vi "Calculate Particle Scores2.vi"(10 "Sorted Data":dbl[][](array[numeric])) -> (3 "Scores":T1[](array[typedef]))   [LabVIEW 2019]
doc: "Calculate scores based on the particle measurements. Calculated scores are for aspect ratio, area to convex hull area, and moment of inertia. These scores range between 0 and 100 and can be used to categorize particles as targets and non-targets."
uses:
  Target Fields.ctl
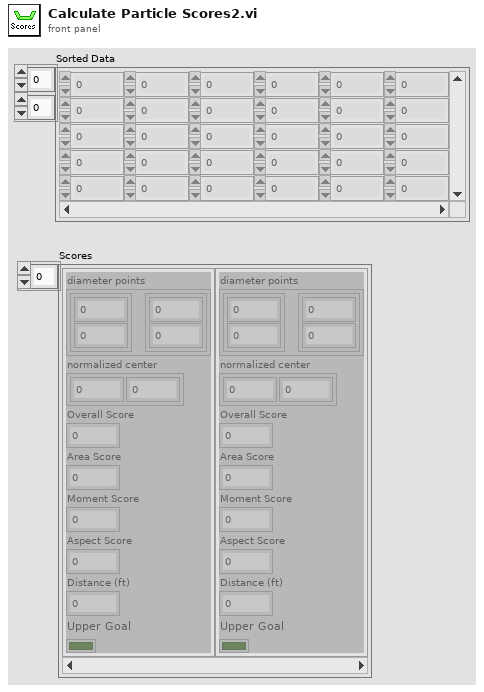
[diagram p1: front panel]
types:
  T1 = typedef "Target Fields.ctl" = cluster{"diameter points":cluster{"first point":cluster{"x":dbl, "y":dbl}, "projected point":cluster{"x":dbl, "y":dbl}}, "normalized center":cluster{"x":dbl, "y":dbl}, "Overall Score":dbl, "Area Score":dbl, "Moment Score":dbl, "Aspect Score":dbl, "Distance (ft)":dbl, "Upper Goal":bool}
  T2 = cluster{cluster{"Numeric":dbl, "Numeric":dbl}, cluster{"Numeric":dbl, "Numeric":dbl}}
  T3 = cluster{"first point":cluster{"x":dbl, "y":dbl}, "projected point":cluster{"x":dbl, "y":dbl}}
  T4 = cluster{cluster{"first point":cluster{"x":dbl, "y":dbl}, "projected point":cluster{"x":dbl, "y":dbl}}, "first point":cluster{"x":dbl, "y":dbl}, dbl, "Score":dbl, "Score":dbl, "Score":dbl, dbl, bool}
  T5 = cluster{cluster{cluster{"Numeric":dbl, "Numeric":dbl}, cluster{"Numeric":dbl, "Numeric":dbl}}, "first point":cluster{"x":dbl, "y":dbl}, dbl, "Score":dbl, "Score":dbl, "Score":dbl, dbl, bool}
  T6 = cluster{cluster{"first point":cluster{"Numeric":dbl, "Numeric":dbl}, "projected point":cluster{"Numeric":dbl, "Numeric":dbl}}, "first point":cluster{"x":dbl, "y":dbl}, dbl, "Score":dbl, "Score":dbl, "Score":dbl, dbl, bool}
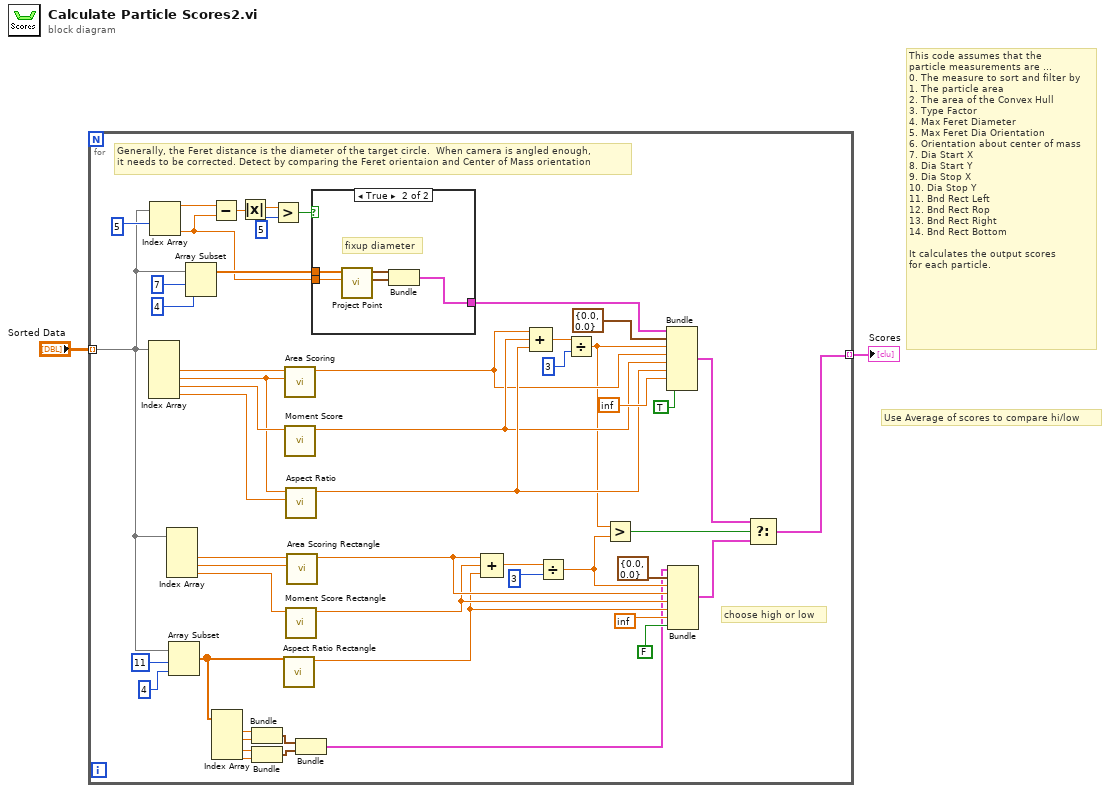
[diagram p0: block diagram]
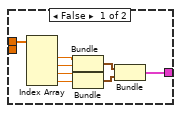
[diagram p2: hidden frame]
diagram:
  # "Use Average of scores to compare hi/low"
  # "This code assumes that the\nparticle measurements are ...\n0. The measure to sort and filter by\n1. The particle area\n2. The area of the Convex Hull\n3. Type Factor\n4. Max Feret Diameter\n5. Max Feret Dia Orientation\n6. Orientation about center of mass\n7. Dia Start X\n8. Dia Start Y\n9. Dia Stop X\n10. Dia Stop Y\n11. Bnd Rect Left\n12. Bnd Rect Rop\n13. Bnd Rect Right\n14. Bnd Rect Bottom\n\nIt calculates the output scores\nfor each particle."
  n1 = for {
    tunnel: "Sorted Data" -> [w27] mode=indexing
    tunnel: [w18] -> w1 mode=indexing
    # "choose high or low"
    # "Generally, the Feret distance is the diameter of the target circle.  When camera is angled enough,\nit needs to be corrected. Detect by comparing the Feret orientaion and Center of Mass orientation"
    n2 = Index Array(array=w27) -> (element #2=w53:dbl, element #3=w51:dbl, element #4=w52:dbl, element #5=w50:dbl)  [unwired: 5 in, 1 out]
    n3 = Index Array(array=w27, index #1=5 ("index")) -> (element #1=w46:dbl, element #2=w41:dbl)  [unwired: 1 in]
    n4 = Index Array(array=w27) -> (element #2=w30:dbl, element #3=w29:dbl, element #4=w28:dbl)  [unwired: 4 in, 1 out]
    n5 = Array Subset(array=w27, index=11, length=4) -> (w10:dbl[])
    n6 = Array Subset(array=w27, index=7, length=4) -> (w42:dbl[])
    n7 = Subtract(x=w46, y=w41) -> (x-y=w49:dbl)
    n8 = Index Array(array=w10) -> (element #1=w9:dbl, element #2=w8:dbl, element #3=w7:dbl, element #4=w6:dbl)  [unwired: 4 in]
    n9 = Absolute Value(x=w49) -> (abs(x)=w47:dbl)
    n10 = Bundle("Numeric"=w9, "Numeric"=w8) -> (w5:cluster{"Numeric":dbl, "Numeric":dbl})  [unwired: 1 in]
    n11 = Bundle("Numeric"=w7, "Numeric"=w6) -> (w4:cluster{"Numeric":dbl, "Numeric":dbl})  [unwired: 1 in]
    n12 = Greater?(x=w47, y=5 ("length")) -> (0:w40:bool)
    n13 = call "Aspect Ratio Rectangle.vi"("Bounds"=w10) -> ("Score"=w13:dbl)  [unwired: 10 in]
    n14 = call "Area Scoring.vi"("Convex Hull Area"=w51, "Area"=w53) -> ("Score"=w34:dbl)  [unwired: 9 in]
    n15 = call "Moment Score.vi"("Moment Factor"=w52) -> ("Score"=w35:dbl)  [unwired: 10 in]
    n16 = call "Aspect Ratio.vi"("Diameter"=w50, "Convex Hull Area"=w51) -> ("Score"=w36:dbl)  [unwired: 9 in]
    n17 = call "Moment Score Rectangle.vi"("Moment Factor"=w28) -> ("Score"=w14:dbl)  [unwired: 10 in]
    n18 = call "Area Scoring Rectangle.vi"("Convex Hull Area"=w29, "Area"=w30) -> ("Score"=w15:dbl)  [unwired: 9 in]
    n19 = Bundle(w5, w4) -> (w3:T2)  [unwired: 1 in]
    n20 = case shown="True" w40 {
      tunnel: w42 -> [w59 w66]
      tunnel: w41 -> [_ w65]
      tunnel: [w54 w62] -> w33
      frame False {
        n21 = Index Array(array=w59) -> (element #1=w57:dbl, element #2=w58:dbl, element #3=w60:dbl, element #4=w61:dbl)  [unwired: 4 in]
        n22 = Bundle("Numeric"=w57, "Numeric"=w58) -> (w56:cluster{"Numeric":dbl, "Numeric":dbl})  [unwired: 1 in]
        n23 = Bundle("Numeric"=w60, "Numeric"=w61) -> (w55:cluster{"Numeric":dbl, "Numeric":dbl})  [unwired: 1 in]
        n24 = Bundle(w56, w55) -> (w54:T2)  [unwired: 1 in]
      }
      frame True {
        # "fixup diameter"
        n25 = call "Project Point.vi"("orientation (deg)"=w65, "coordinates"=w66) -> ("projected point"=w63:cluster{"x":dbl, "y":dbl}, "first point"=w64:cluster{"x":dbl, "y":dbl})  [unwired: 8 in]
        n26 = Bundle("first point"=w64, "projected point"=w63) -> (w62:T3)  [unwired: 1 in]
      }
    }
    n27 = Compound Arithmetic op=ADD(w15, w14, w13) -> (w24:dbl)
    n28 = Compound Arithmetic op=ADD(w34, w35, w36) -> (w38:dbl)
    n29 = Divide(x=w24, y=3) -> (x/y=w16:dbl)
    n30 = Divide(x=w38, y=3) -> (x/y=w22:dbl)
    n31 = Greater?(x=w22, y=w16) -> (0:w21:bool)
    n32 = Bundle(w33, "first point"=cluster{"x":dbl, "y":dbl} {"x"=0.0, "y"=0.0}, w22, "Score"=w34, "Score"=w35, "Score"=w36, inf, TRUE) -> (w19:T4)  [unwired: 1 in]
    n33 = Bundle(w3, "first point"=cluster{"x":dbl, "y":dbl} {"x"=0.0, "y"=0.0}, w16, "Score"=w15, "Score"=w14, "Score"=w13, inf, FALSE) -> (w20:T5)  [unwired: 1 in]
    n34 = Select(t=w19, s=w21, f=w20) -> (s? t:f=w18:T6)
  }
  "Scores" <- w1
